vi "Parse Float.vi"(8 "error in (no error)":errorcluster, 11 "Alpaca CLI Parser in":refnum<class "JSON Parser.lvclass">) -> (0 "error out":errorcluster, 2 "Value":variant, 3 "Alpaca CLI Parser out":refnum<class "JSON Parser.lvclass">)   [LabVIEW 2020, in "JKI JSON Serialization.lvlib" / "JSON Parser.lvclass"]
uses:
  JSON Parser.lvclass
  C:/Users/nate/Documents/JKI-JSON-Serialization/src/Deserializer/Parser/Parser.lvclass
  Parser/Parser.lvclass/Parser.ctl
  Parser/Lookahead.vi
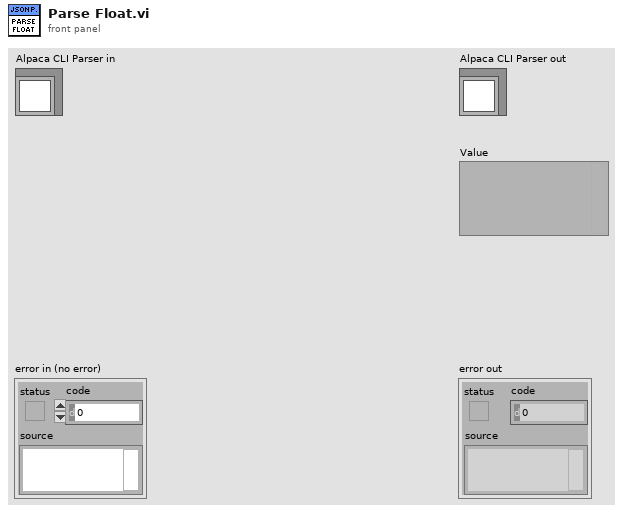
[diagram p1: front panel]
types:
  T1 = typedef "JKI JSON Serialization.lvlib/JSON Lexer.lvclass/JSON Token Type.ctl" = enum32{"unknown", "comma", "end-label", "begin-object", "end-object", "begin-array", "end-array", "quoted-string", "boolean", "exponential-number", "decimal-number", "integer-number", "special-number", "null", "symbol", "whitespace", "EOF"}
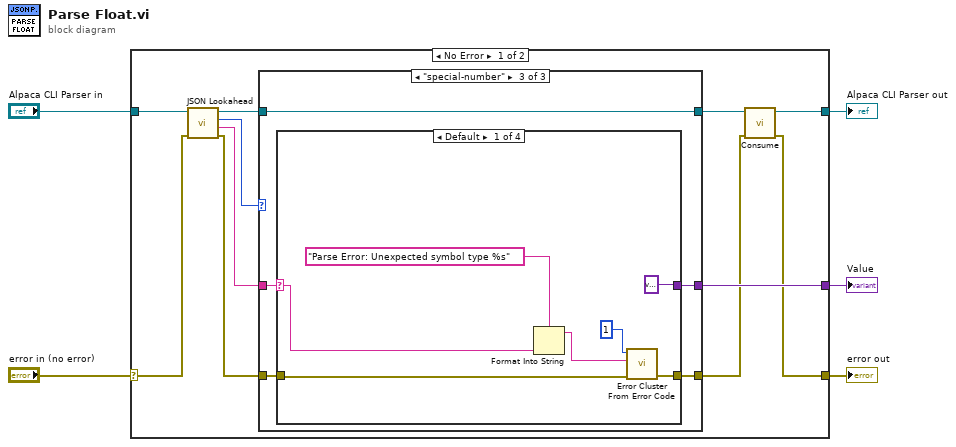
[diagram p0: block diagram]
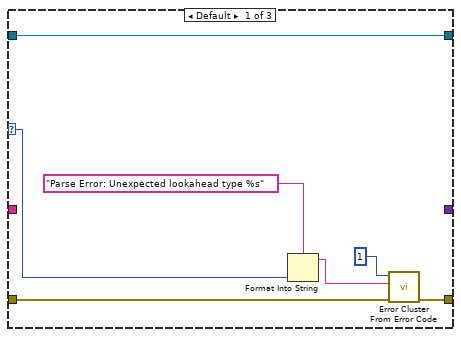
[diagram p2: hidden frame]
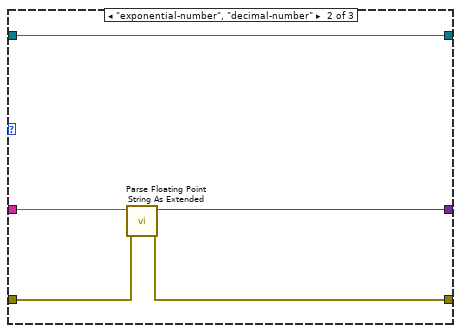
[diagram p3: hidden frame]
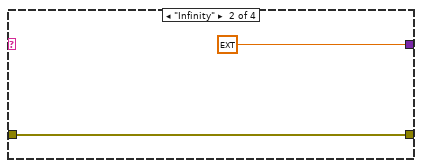
[diagram p4: hidden frame]
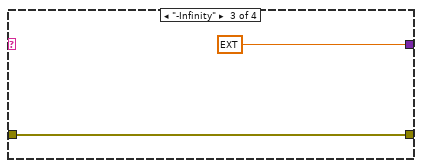
[diagram p5: hidden frame]
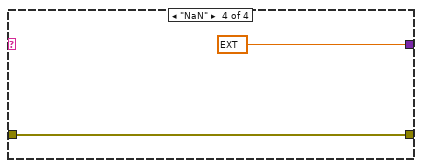
[diagram p6: hidden frame]
diagram:
  n1 = case shown="No Error" "error in (no error)" {
    selector: "error in (no error)" -> [w15 w48]
    tunnel: [w7 w48] -> w4
    tunnel: [w8 w47] -> w2
    tunnel: "Alpaca CLI Parser in" -> [w16 w47]
    tunnel: [w10 _] -> w1
    frame No Error {
      n2 = call "JSON Lookahead.vi"("error in (no error)"=w15, "Alpaca CLI Parser in"=w16) -> ("error out"=w12:errorcluster, "Lookahead Value"=w11:string, "Lookahead Type"=w13:T1, "Alpaca CLI Parser out"=w14:refnum<class "JSON Parser.lvclass">)  [unwired: 6 in]
      n3 = case shown="\"special-number\"" w13 {
        selector: w13 -> [w19 _ _]
        tunnel: w14 -> [w17 w24 w33]
        tunnel: [w17 w24 w33] -> w9
        tunnel: [w23 w25 w29] -> w6
        tunnel: w12 -> [w22 w27 w31]
        tunnel: w11 -> [_ w28 w32]
        tunnel: [_ w26 w30] -> w10
        frame Default {
          n4 = Format Into String(format string="Parse Error: Unexpected lookahead type %s" ("error message (\"\")"), w19) -> (resulting string=w18:string)  [unwired: 2 in, 1 out]
          n5 = call <vilib>:"Error Cluster From Error Code.vi"("error in (no error)"=w22, "error message (\"\")"=w18, "error code (0)"=1) -> ("error out"=w23:errorcluster)  [unwired: 6 in]
        }
        frame "exponential-number", "decimal-number" {
          n6 = call "Parse Floating Point String As Extended.vi"("error in (no error)"=w27, "String"=w28) -> ("error out"=w25:errorcluster, "Value"=w26:variant)  [unwired: 8 in]
        }
        frame "special-number" {
          n7 = case shown="Default" w32 {
            selector: w32 -> [w37 _ _ _]
            tunnel: w31 -> [w35 w41 w43 w45]
            tunnel: [variant ext inf ext -inf ext nan] -> w30
            tunnel: [w36 w41 w43 w45] -> w29
            frame Default {
              n8 = Format Into String(format string="Parse Error: Unexpected symbol type %s" ("error message (\"\")"), w37) -> (resulting string=w38:string)  [unwired: 2 in, 1 out]
              n9 = call <vilib>:"Error Cluster From Error Code.vi"("error in (no error)"=w35, "error message (\"\")"=w38, "error code (0)"=1) -> ("error out"=w36:errorcluster)  [unwired: 6 in]
            }
            frame "Infinity" {
            }
            frame "-Infinity" {
            }
            frame "NaN" {
            }
          }
        }
      }
      n10 = call-dynamic "Consume.vi"("error in (no error)"=w6, "Alpaca Parser in"=w9) -> ("error out"=w7:errorcluster, "Alpaca Parser out"=w8:refnum<class "JSON Parser.lvclass">)  [unwired: 8 in]
    }
    frame Error {
    }
  }
  "error out" <- w4
  "Alpaca CLI Parser out" <- w2
  "Value" <- w1
